vi "svx_DUT.vi"(0 "Stimulus":waveform(dbl), 5 "error in (no error)":errorcluster, 7 "DUT":T1(ring), 9 "Fc":dbl=1000.0 format="%.2f") -> (14 "dup Stimulus":waveform(dbl), 15 "response signal Y [EUy]":waveform(dbl), 19 "error out":errorcluster)   [LabVIEW 2017]
doc: "Inserts DUT (digital filter) into signal path. Stimulus is returned unchanged. Response is the filtered signal."
uses:
  <vilib>/measure/macond.llb/IIR Filter for 1 Chan.vi
  <vilib>/measure/macond.llb/FIR Filter for 1 Chan.vi
  <vilib>/measure/NI_MAPro.lvlib
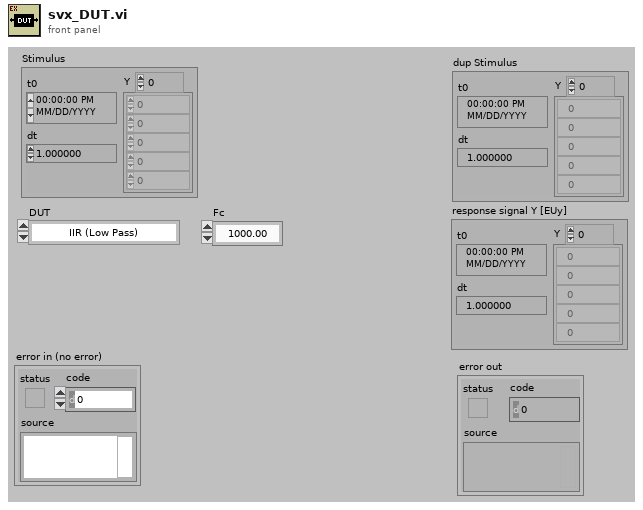
[diagram p1: front panel]
types:
  T1 = enum16{"IIR (Low Pass)", "IIR (Band Pass)", "FIR (Low pass - 50 Taps)", "Notch filter"}
  T2 = cluster{"Topology":enum16{"Off", "Butterworth", "Chebyshev", "Inverse Chebyshev", "Elliptic", "Bessel"}, "Type":enum16{"Lowpass", "Highpass", "Bandpass", "Bandstop"}, "Order":i32, "Lower Fc":dbl, "Upper Fc":dbl, "PB Ripple":dbl, "SB Attenuation":dbl}
  T3 = cluster{"Topology":enum16{"Off", "FIR by Specification", "Equi-ripple FIR", "Windowed FIR"}, "Type":enum16{"Lowpass", "Highpass", "Bandpass", "Bandstop"}, "#Taps":i32, "Lower PB":dbl, "Upper PB":dbl, "Lower SB":dbl, "Upper SB":dbl}
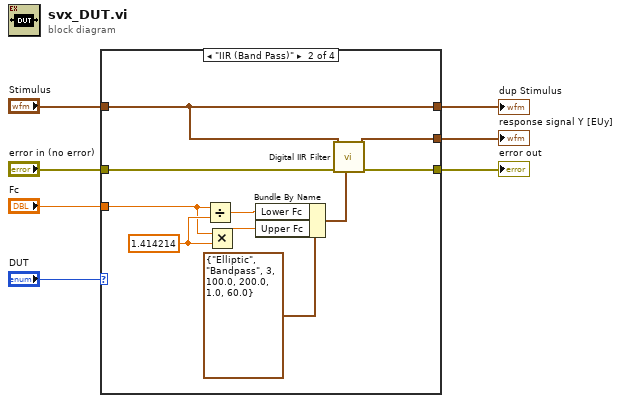
[diagram p0: block diagram]
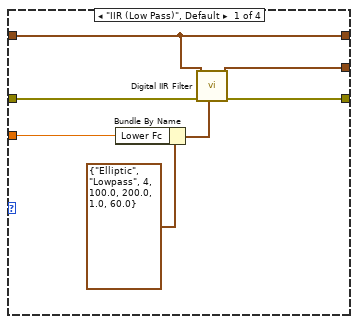
[diagram p2: hidden frame]
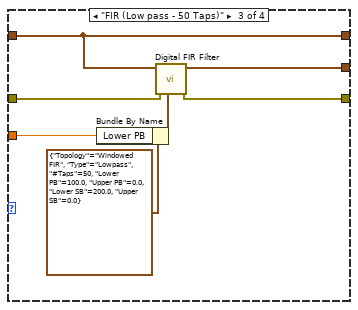
[diagram p3: hidden frame]
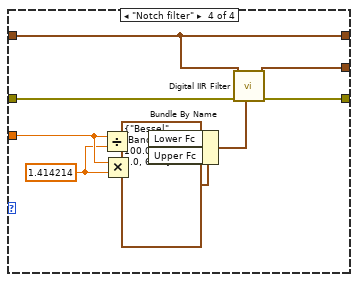
[diagram p4: hidden frame]
diagram:
  n1 = case shown="\"IIR (Band Pass)\"" "DUT" {
    tunnel: [w14 w23 w28 w38] -> w7
    tunnel: "Stimulus" -> [w8 w19 w30 w41]
    tunnel: [w13 w22 w31 w39] -> w6
    tunnel: "error in (no error)" -> [w12 w24 w29 w40]
    tunnel: "Fc" -> [w9 w17 w27 w34]
    tunnel: [w8 w19 w30 w41] -> w1
    frame "IIR (Low Pass)", Default {
      n2 = Bundle By Name(cluster=T2 {"Topology"=enum."Elliptic", "Type"=enum."Lowpass", "Order"=4, "Lower Fc"=100.0, "Upper Fc"=200.0, "PB Ripple"=1.0, "SB Attenuation"=60.0} ("IIR filter specifications"), "Lower Fc"=w9) -> (w10:T2)
      n3 = call-poly <vilib>:"Digital IIR Filter.vi"("IIR filter specifications"=w10, "error in (no error)"=w12, "signal in"=w8) -> ("error out"=w14:errorcluster, "signal out"=w13:waveform(dbl))  [unwired: 6 in, 1 out]
    }
    frame "IIR (Band Pass)" {
      w18 = 1.414214 ("sqrt(x)")
      n4 = Divide(x=w17, y=w18) -> (x/y=w16:dbl)
      n5 = Multiply(x=w17, y=w18) -> (x*y=w15:dbl)
      n6 = Bundle By Name(cluster=T2 {"Topology"=enum."Elliptic", "Type"=enum."Bandpass", "Order"=3, "Lower Fc"=100.0, "Upper Fc"=200.0, "PB Ripple"=1.0, "SB Attenuation"=60.0} ("IIR filter specifications"), "Lower Fc"=w16, "Upper Fc"=w15) -> (w20:T2)
      n7 = call-poly <vilib>:"Digital IIR Filter.vi"("IIR filter specifications"=w20, "error in (no error)"=w24, "signal in"=w19) -> ("error out"=w23:errorcluster, "signal out"=w22:waveform(dbl))  [unwired: 6 in, 1 out]
    }
    frame "FIR (Low pass - 50 Taps)" {
      n8 = Bundle By Name(cluster=T3 {"Topology"=enum."Windowed FIR", "Type"=enum."Lowpass", "#Taps"=50, "Lower PB"=100.0, "Upper PB"=0.0, "Lower SB"=200.0, "Upper SB"=0.0} ("FIR filter specifications"), "Lower PB"=w27) -> (w25:T3)
      n9 = call-poly <vilib>:"Digital FIR Filter.vi"("FIR filter specifications"=w25, "error in (no error)"=w29, "signal in"=w30) -> ("error out"=w28:errorcluster, "signal out"=w31:waveform(dbl))  [unwired: 6 in, 1 out]
    }
    frame "Notch filter" {
      w33 = 1.414214 ("sqrt(x)")
      n10 = Divide(x=w34, y=w33) -> (x/y=w32:dbl)
      n11 = Multiply(x=w34, y=w33) -> (x*y=w35:dbl)
      n12 = Bundle By Name(cluster=T2 {"Topology"=enum."Bessel", "Type"=enum."Bandstop", "Order"=3, "Lower Fc"=100.0, "Upper Fc"=200.0, "PB Ripple"=1.0, "SB Attenuation"=60.0} ("IIR filter specifications"), "Lower Fc"=w32, "Upper Fc"=w35) -> (w36:T2)
      n13 = call-poly <vilib>:"Digital IIR Filter.vi"("IIR filter specifications"=w36, "error in (no error)"=w40, "signal in"=w41) -> ("error out"=w38:errorcluster, "signal out"=w39:waveform(dbl))  [unwired: 6 in, 1 out]
    }
  }
  "error out" <- w7
  "response signal Y [EUy]" <- w6
  "dup Stimulus" <- w1
